vi "Save.vi"(8 "error in (no error)":errorcluster, 10 "Path":path, 11 "Collection in":refnum<class "Collection.lvclass">) -> (0 "error out":errorcluster, 3 "Collection out":refnum<class "Collection.lvclass">)   [LabVIEW 2021, in "LvMarkdown.lvlib" / "Collection.lvclass"]
uses:
  Collection.lvclass
  Collection.lvclass/Collection.ctl
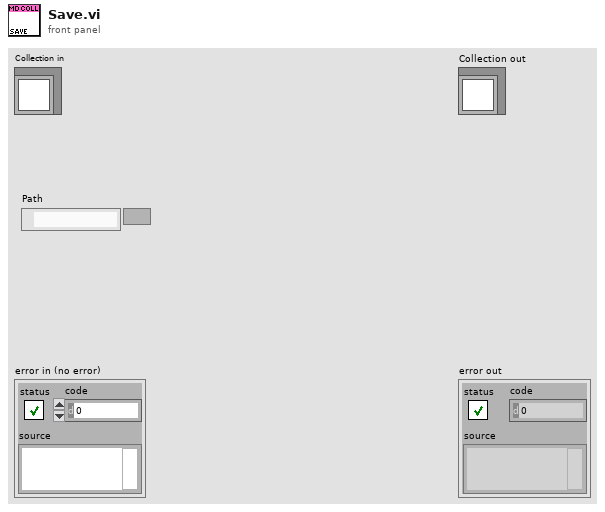
[diagram p1: front panel]
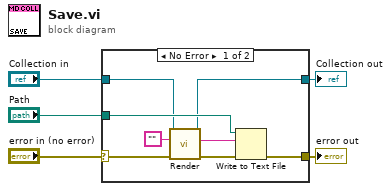
[diagram p0: block diagram]
diagram:
  n1 = case shown="No Error" "error in (no error)" {
    selector: "error in (no error)" -> [w7 w15]
    tunnel: [w10 w15] -> w4
    tunnel: [w9 w14] -> w2
    tunnel: "Collection in" -> [w8 w14]
    tunnel: "Path" -> [w11 _]
    frame No Error {
      n2 = call-dynamic "Render.vi"("error in (no error)"=w7, "String in"="", "Collection in"=w8) -> ("error out"=w6:errorcluster, "String out"=w13:string, "Collection out"=w9:refnum<class "Collection.lvclass">)  [unwired: 6 in]
      n3 = Write to Text File(file (use dialog)=w11, text=w13, error in=w6) -> (error out=w10:errorcluster)  [unwired: 1 in, 2 out]
    }
    frame Error {
    }
  }
  "error out" <- w4
  "Collection out" <- w2
